vi "Launch Plugin (Path).vi"(8 "error in (no error)":errorcluster, 10 "Path":path, 11 "GUI Manager Module in":refnum<class "GUI Manager Module.lvclass">) -> (0 "error out":errorcluster, 3 "GUI Manager Module out":refnum<class "GUI Manager Module.lvclass">)   [LabVIEW 2020, in "VolatusGUI.lvlib" / "GUI Manager Module.lvclass"]
uses:
  GUI Manager Module.lvclass
  C:/dev/lv20CE/relink/lv-volatus/Volatus/Module/Module.lvclass
  VolatusConfig/VolatusConfigElement/VolatusConfigElement.lvclass
  PluginGUI/PluginGUI.lvclass
  GUI Manager Module.lvclass/GUI Manager Module.ctl
  Volatus/Module/Module.lvclass
  Volatus/Volatus.lvlib
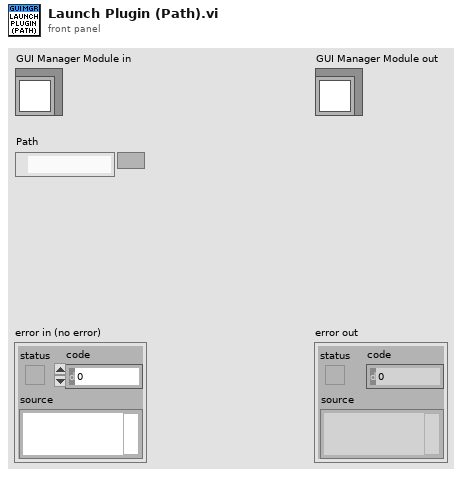
[diagram p1: front panel]
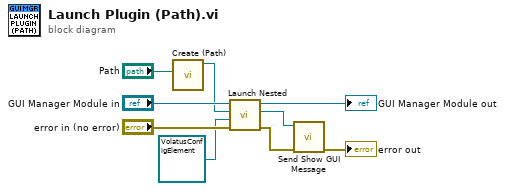
[diagram p0: block diagram]
diagram:
  n1 = call "Create (Path).vi"("Plugin GUI Path"="Path") -> ("PluginGUI out"=w4:refnum<class "PluginGUI.lvclass">)  [unwired: 9 in, 1 out]
  n2 = call "Launch Nested.vi"("error in (no error)"="error in (no error)", "Config Element"=refnum<class "VolatusConfigElement.lvclass"> refnum, "Nested Module"=w4, "Parent in"="GUI Manager Module in") -> ("error out"=w2:errorcluster, "MessageQ"=w3:refnum<class "MessageQ.lvclass">, "Parent out"=→"GUI Manager Module out":refnum<class "GUI Manager Module.lvclass">)  [unwired: 5 in]
  n3 = call "Send Show GUI Message.vi"("error in (no error)"=w2, "MessageQ"=w3) -> ("error out"=→"error out":errorcluster)  [unwired: 9 in]
